vi "OAT Waterfall Configure Plots Color.vi"(4 "# of axis lines":i32, 5 "color changed?":bool, 6 "# of grid lines":i32, 7 "BG color":u32(colorbox)=65280, 8 "# of new spectra":i32, 9 "Num of displayed spectra":i32, 10 "plot settings":T1={"plot color"=0, "grid color"=0, "X shift (rel to total X)"=0.1, "max Z range"=11, "number of spectra"=40} {"max Z range" items=["10^-7", "10^-6", "10^-5", "0.0001", "0.001", "0.01", "0.1", "1", "10", "100", "1000", "auto z range"]; "X shift (rel to total X)" format="%.2f"}, 11 "reference":refnum<vi>) -> (3 "reference out":refnum<vi>)   [LabVIEW 2017]
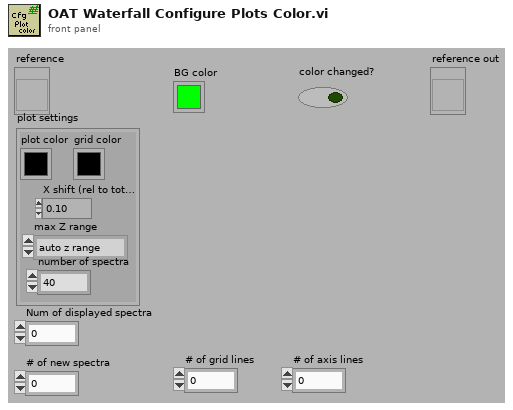
[diagram p1: front panel]
types:
  T1 = cluster{"plot color":u32, "grid color":u32, "X shift (rel to total X)":dbl, "max Z range":u16, "number of spectra":i32}
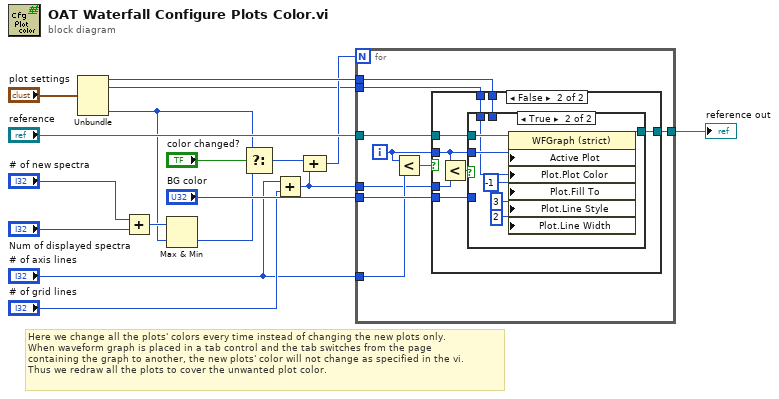
[diagram p0: block diagram]
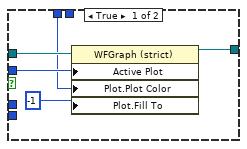
[diagram p2: hidden frame]
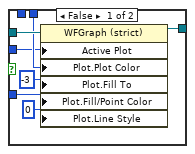
[diagram p3: hidden frame]
diagram:
  # "Here we change all the plots' colors every time instead of changing the new plots only.\nWhen waveform graph is placed in a tab control and the tab switches from the page\ncontaining the graph to another, the new plots' color will not change as specified in the vi.\nThus we redraw all the plots to cover the unwanted plot color."
  n1 = Unbundle("plot settings") -> ("plot color"=w7:u32, "grid color"=w4:u32, "number of spectra"=w3:i32)  [unwired: 2 out]
  n2 = Add(x="# of new spectra", y="Num of displayed spectra") -> (x+y=w10:i32)
  n3 = Max & Min(x=w10, y=w3) -> (min(x,y)=w9:i32)  [unwired: 1 out]
  n4 = Select(t=w3, s="color changed?", f=w9) -> (s? t:f=w14:i32)
  n5 = Add(x="# of axis lines", y="# of grid lines") -> (x+y=w1:i32)
  n6 = Compound Arithmetic op=ADD(w14, w1) -> (w5:i32)
  n7 = for {
    N: w5 -> [_]
    tunnel: "reference" -> [w26]
    tunnel: "BG color" -> [w25]
    tunnel: w7 -> [w24]
    tunnel: [w23] -> w8
    tunnel: w4 -> [w20]
    tunnel: "# of axis lines" -> [w19]
    tunnel: w1 -> [w18]
    i -> [w22]
    n8 = Less?(x=w22, y=w19) -> (x < y?=w21:bool)
    n9 = case shown="False" w21 {
      tunnel: w26 -> [w31 w39]
      tunnel: w25 -> [_ w38]
      tunnel: w24 -> [_ w37]
      tunnel: [w29 w36] -> w23
      tunnel: w22 -> [w28 w35]
      tunnel: w20 -> [w27 w32]
      tunnel: w18 -> [_ w34]
      frame True {
        n10 = property on="Property Node" class="WFGraph (strict)"(reference=w31, "Active Plot"=w28, "Plot.Plot Color"=w27, "Plot.Fill To"=i16 -1) -> (reference out=w29:refnum<vi>)  [unwired: 1 in, 1 out]
      }
      frame False {
        n11 = Less?(x=w35, y=w34) -> (x < y?=w33:bool)
        n12 = case shown="True" w33 {
          tunnel: w39 -> [w46 w51]
          tunnel: w38 -> [w44 _]
          tunnel: w37 -> [w43 _]
          tunnel: [w42 w50] -> w36
          tunnel: w35 -> [w41 w52]
          tunnel: w32 -> [_ w49]
          frame False {
            n13 = property on="Property Node" class="WFGraph (strict)"(reference=w46, "Active Plot"=w41, "Plot.Plot Color"=w43, "Plot.Fill To"=i16 -3, "Plot.Fill/Point Color"=w44, "Plot.Line Style"=u8 0) -> (reference out=w42:refnum<vi>)  [unwired: 1 in, 1 out]
          }
          frame True {
            n14 = property on="Property Node" class="WFGraph (strict)"(reference=w51, "Active Plot"=w52, "Plot.Plot Color"=w49, "Plot.Fill To"=i16 -1, "Plot.Line Style"=u8 3, "Plot.Line Width"=u8 2) -> (reference out=w50:refnum<vi>)  [unwired: 1 in, 1 out]
          }
        }
      }
    }
  }
  "reference out" <- w8
